vi "upper_test_section_pressure.vi"(2 "Offset [Pa]":dbl, 4 "Waveform Graph":dynamicdata(graph)) -> (0 "Offset Absolute Pressure [Pa]":dbl, 1 "Absolute Pressure [Pa]":dbl)   [LabVIEW 2015]
uses:
  <vilib>/express/express arith-compare/Formula/XNode/ExpressFormulaBlockNode.xnode
  <vilib>/express/express shared/transition.llb/Dynamic To Waveform Array.vi
  <vilib>/express/express arith-compare/Formula/Block/exnFormulaBlock how many pts in the wave.vi
  <vilib>/express/express shared/ex_Modify Signal Name.vi
  <vilib>/express/express shared/transition.llb/Waveform Array To Dynamic.vi
panel:
  in  "Abs. Pressure\nVoltage [V]":dbl
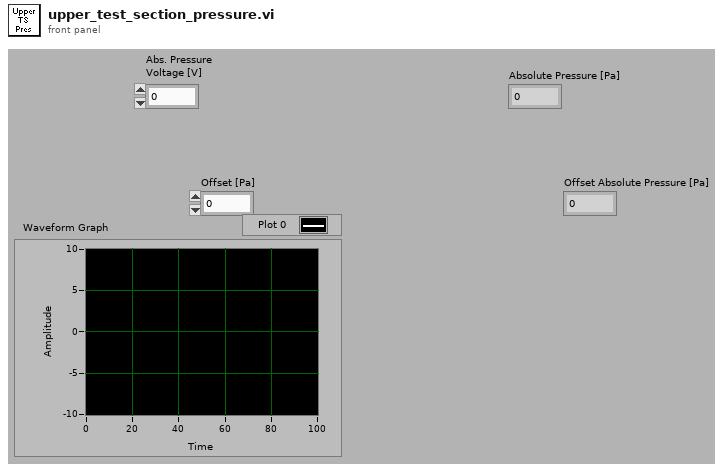
[diagram p1: front panel]
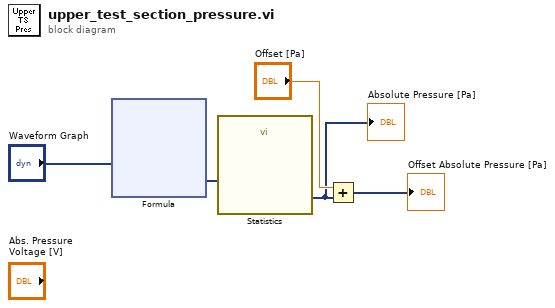
[diagram p0: block diagram]
diagram:
  n1 = xnode "Formula"("V"="Waveform Graph") -> ("Result"=w5:dynamicdata)  [unwired: 1 in, 1 out]
  n2 = call "Statistics"("Signals"=w5) -> ("Arithmetic Mean"=w2:dynamicdata)  [unwired: 25 in, 1 out]
  "Absolute Pressure [Pa]" <- w2
  n3 = Add(x="Offset [Pa]", y=w2) -> (x+y=→"Offset Absolute Pressure [Pa]":dynamicdata)
